vi "Parameters to Front Panel.vi"(8 "error in (no error)":errorcluster, 11 "Mag Lab Root in":refnum<class "Mag Lab Root.lvclass">) -> (0 "error out":errorcluster, 3 "Mag Lab Root out":refnum<class "Mag Lab Root.lvclass">)   [LabVIEW 2015, in "Mag Lab Root.lvclass"]
uses:
  Mag Lab Root.lvclass
  Mag Lab Properties/Mag Lab Parameters.lvclass
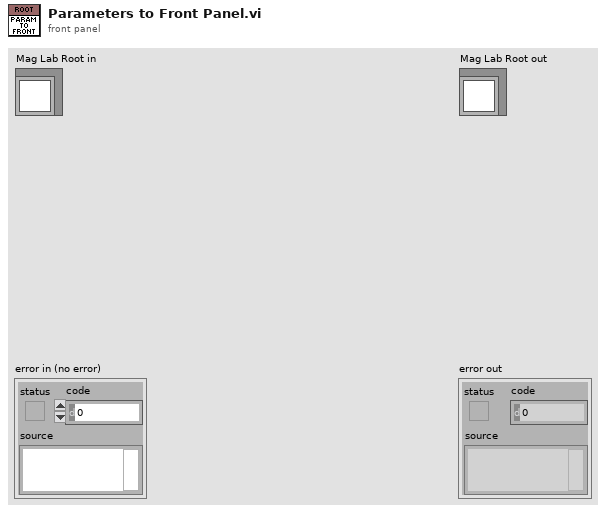
[diagram p1: front panel]
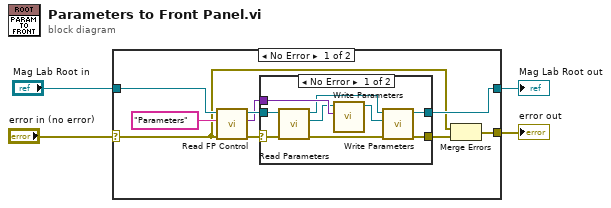
[diagram p0: block diagram]
diagram:
  n1 = case shown="No Error" "error in (no error)" {
    selector: "error in (no error)" -> [w6 w25]
    tunnel: [w5 w25] -> w3
    tunnel: [w7 w24] -> w1
    tunnel: "Mag Lab Root in" -> [w8 w24]
    frame No Error {
      n2 = call-dynamic "Read FP Control.vi"("error in (no error)"=w6, "Control Name"="Parameters", "Mag Lab Root in"=w8) -> ("error out"=w10:errorcluster, "Control Value"=w11:variant, "Mag Lab Root out"=w12:refnum<class "Mag Lab Root.lvclass">)  [unwired: 6 in]
      n3 = case shown="No Error" w10 {
        selector: w10 -> [w15 _]
        tunnel: w11 -> [w20 _]
        tunnel: w12 -> [w18 w23]
        tunnel: [w22 _] -> w13
        tunnel: [w21 w23] -> w7
        frame No Error {
          n4 = call-dynamic "Read Parameters.vi"("error in (no error)"=w15, "Mag Lab Root in"=w18) -> ("error out"=w14:errorcluster, "Mag Lab Parameters.lvclass"=w16:refnum<class "Mag Lab Parameters.lvclass">, "Mag Lab Root out"=w17:refnum<class "Mag Lab Root.lvclass">)  [unwired: 7 in]
          n5 = call-dynamic "Write Parameters.vi"("Parameters"=w20, "Mag Lab Parameters in"=w16) -> ("Mag Lab Parameters out"=w19:refnum<class "Mag Lab Parameters.lvclass">)  [unwired: 8 in, 1 out]
          n6 = call-dynamic "Write Parameters.vi"("error in (no error)"=w14, "Mag Lab Parameters.lvclass"=w19, "Mag Lab Root in"=w17) -> ("error out"=w22:errorcluster, "Mag Lab Root out"=w21:refnum<class "Mag Lab Root.lvclass">)  [unwired: 7 in]
        }
        frame Error {
        }
      }
      n7 = Merge Errors(w6, w13) -> (w5:errorcluster)
    }
    frame Error {
    }
  }
  "error out" <- w3
  "Mag Lab Root out" <- w1
